vi "geve-parse_read_buffer.vi"(8 "error in (no error)":errorcluster, 11 "Runtime Data in":T1) -> (0 "error out":errorcluster, 3 "Runtime Data out":T1)   [LabVIEW 2018]
doc: "convert the raw read buffer into relevant data following the scheme defined."
uses:
  geve-runtime_data_cluster.ctl
  geve-monitoring_data_cluster.ctl
  geve-serial_config_cluster.ctl
  geve-com_ref_cluster.ctl
  geve-message_cluster.ctl
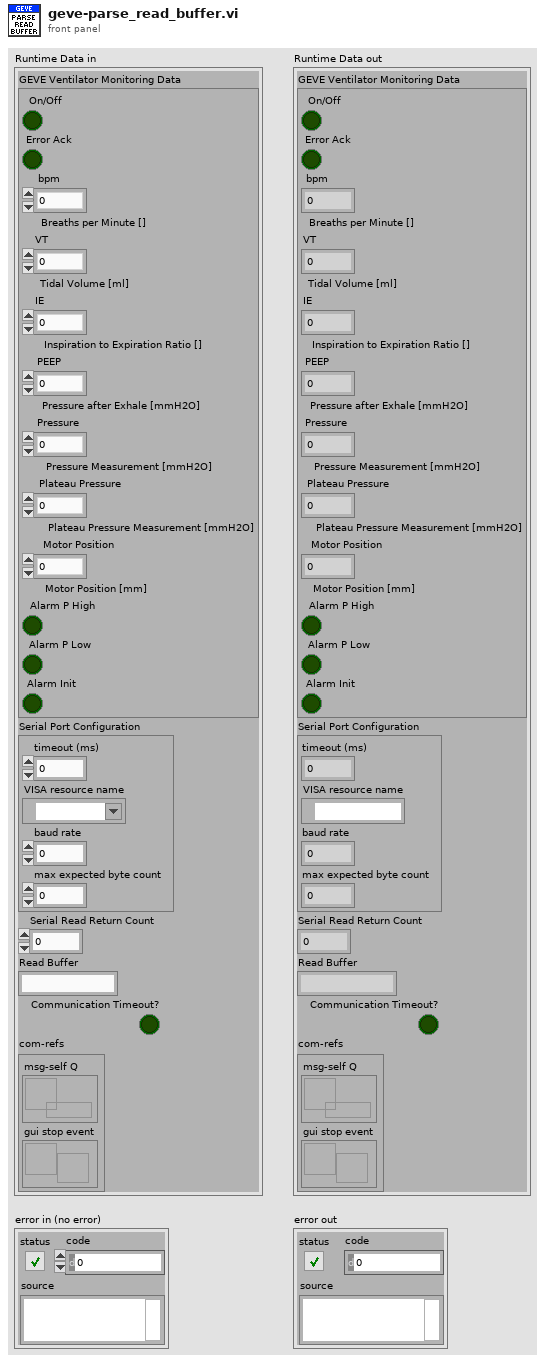
[diagram p1: front panel]
types:
  T1 = typedef "geve-runtime_data_cluster.ctl" = cluster{"GEVE Ventilator Monitoring Data":T2, "Serial Port Configuration":T3, "Serial Read Return Count":u32, "Read Buffer":string, "Communication Timeout?":bool, "com-refs":T4}
  T2 = typedef "geve-monitoring_data_cluster.ctl" = cluster{"On/Off":bool, "Error Ack":bool, "bpm":dbl, "VT":dbl, "IE":dbl, "PEEP":dbl, "Pressure":dbl, "Plateau Pressure":dbl, "Motor Position":dbl, "Alarm P High":bool, "Alarm P Low":bool, "Alarm Init":bool}
  T3 = typedef "geve-serial_config_cluster.ctl" = cluster{"timeout (ms)":u32, "VISA resource name":refnum<visa-resource-name>, "baud rate":u32, "max expected byte count":u32}
  T4 = typedef "geve-com_ref_cluster.ctl" = cluster{"msg-self Q":refnum<queue>, "gui stop event":refnum<user-event>}
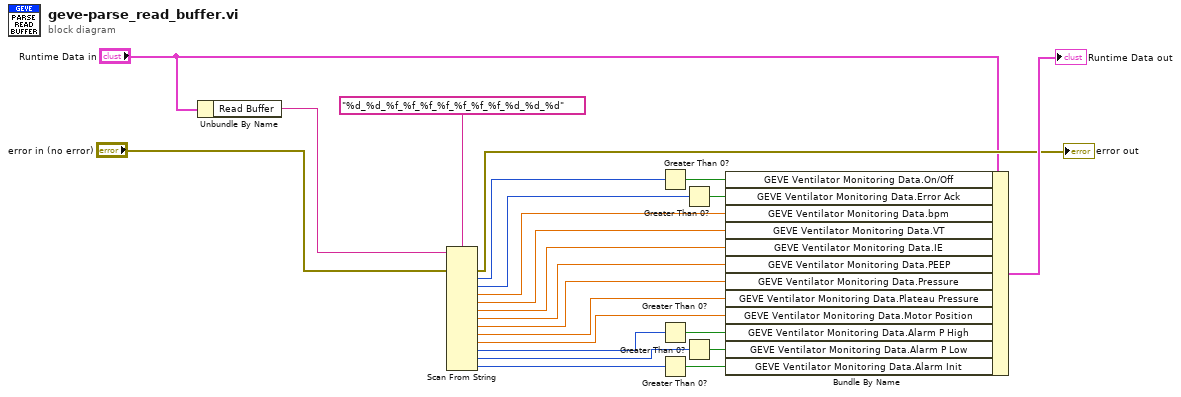
[diagram p0: block diagram]
diagram:
  n1 = Unbundle By Name("Runtime Data in") -> ("Read Buffer"=w20:string)
  n2 = Scan From String(format string="%d_%d_%f_%f_%f_%f_%f_%f_%f_%d_%d_%d", input string=w20, error in="error in (no error)") -> (error out=→"error out":errorcluster, output 1=w18:i32, output 2=w17:i32, output 3=w2:dbl, output 4=w3:dbl, output 5=w4:dbl, output 6=w5:dbl, output 7=w13:dbl, output 8=w14:dbl, output 9=w9:dbl, output 10=w10:i32, output 11=w11:i32, output 12=w12:i32)  [unwired: 13 in, 2 out]
  n3 = Greater Than 0?(x=w18) -> (x > 0?=w16:bool)
  n4 = Greater Than 0?(x=w10) -> (x > 0?=w6:bool)
  n5 = Greater Than 0?(x=w12) -> (x > 0?=w8:bool)
  n6 = Greater Than 0?(x=w17) -> (x > 0?=w15:bool)
  n7 = Greater Than 0?(x=w11) -> (x > 0?=w7:bool)
  n8 = Bundle By Name(cluster="Runtime Data in", "GEVE Ventilator Monitoring Data.On/Off"=w16, "GEVE Ventilator Monitoring Data.Error Ack"=w15, "GEVE Ventilator Monitoring Data.bpm"=w2, "GEVE Ventilator Monitoring Data.VT"=w3, "GEVE Ventilator Monitoring Data.IE"=w4, "GEVE Ventilator Monitoring Data.PEEP"=w5, "GEVE Ventilator Monitoring Data.Pressure"=w13, "GEVE Ventilator Monitoring Data.Plateau Pressure"=w14, "GEVE Ventilator Monitoring Data.Motor Position"=w9, "GEVE Ventilator Monitoring Data.Alarm P High"=w6, "GEVE Ventilator Monitoring Data.Alarm P Low"=w7, "GEVE Ventilator Monitoring Data.Alarm Init"=w8) -> (→"Runtime Data out":T1)
